vi "AUTOFOCUS_automatic_detection.vi"(0 "X array":dbl[](array[numeric]), 1 "QPD array":dbl[](array[numeric]), 2 "Stage type":string, 5 "QPD ref":T1, 7 "Slope":dbl, 9 "QPD":T1, 11 "error in":errorcluster, 12 "Search array":dbl[](array[numeric])) -> (3 "QPD array out":dbl[](array[numeric]), 4 "X array out":dbl[](array[numeric]), 6 "Cursor":cluster{"X":dbl, "Y":dbl}, 8 "Setpoint detected":bool, 10 "norm":dbl, 15 "error out":errorcluster)   [LabVIEW 2015]
uses:
  <vilib>/Analysis/_algsub.llb/Vector Norm Type.ctl
  <vilib>/Analysis/_algsub.llb/Real Vector Norm.vi
  <vilib>/Analysis/NI_AAL_SigProc.lvlib
  <vilib>/Analysis/NI_AALPro.lvlib
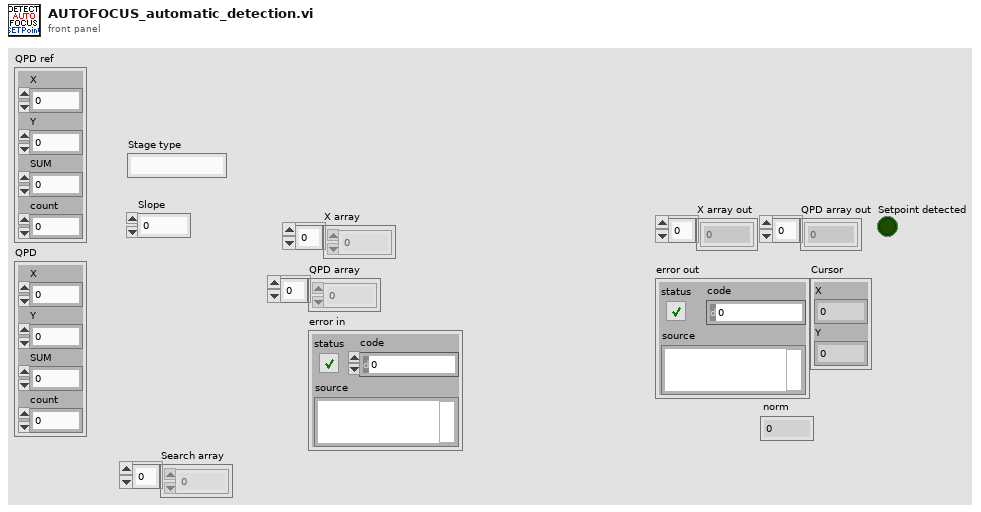
[diagram p1: front panel]
types:
  T1 = cluster{"X":sgl, "Y":sgl, "SUM":sgl, "count":u32}
  T2 = typedef "NI_AALPro.lvlib/Vector Norm Type.ctl" = u16
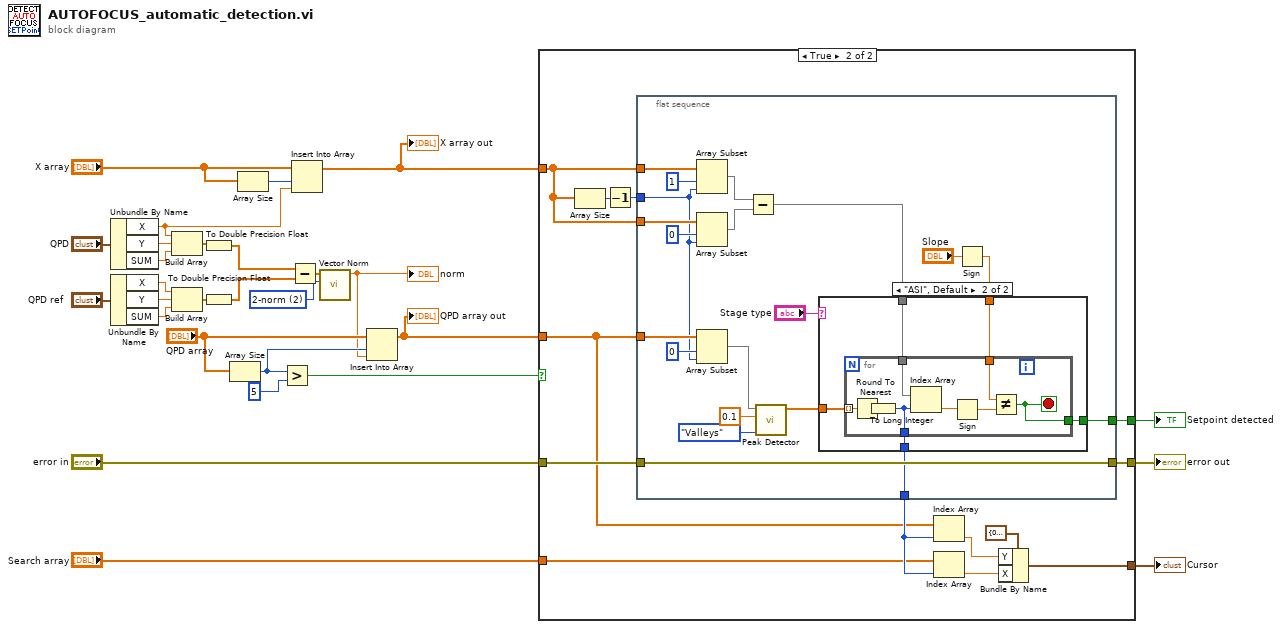
[diagram p0: block diagram]
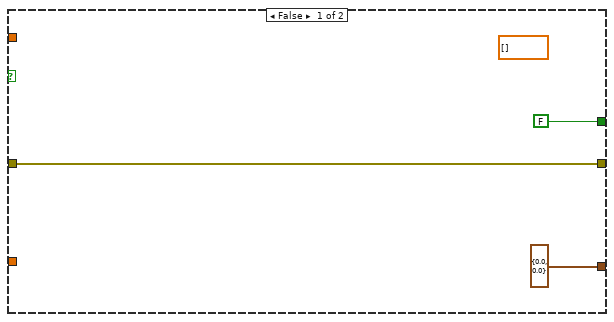
[diagram p2: hidden frame]
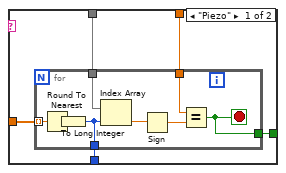
[diagram p3: hidden frame]
diagram:
  w18 = T2 2 items=["1-norm"=1, "2-norm"=2, "Inf-norm"=3, "-Inf-norm"=4, "User Defined"=5] ("norm type")
  n1 = Unbundle By Name("QPD") -> ("X"=w3:sgl, "Y"=w12:sgl, "SUM"=w11:sgl)
  n2 = Unbundle By Name("QPD ref") -> ("X"=w6:sgl, "Y"=w8:sgl, "SUM"=w9:sgl)
  n3 = Build Array(w3, w12, w11) -> (w10:sgl[])
  n4 = Build Array(w6, w8, w9) -> (w7:sgl[])
  n5 = To Double Precision Float(number=w10) -> (double precision float=w2:dbl[])
  n6 = To Double Precision Float(number=w7) -> (double precision float=w1:dbl[])
  n7 = Array Size(array="QPD array") -> (size(s)=w16:i32)
  n8 = Array Size(array="X array") -> (size(s)=w22:i32)
  n9 = Greater?(x=w16, y=5) -> (0:w27:bool)
  n10 = Subtract(x=w2, y=w1) -> (x-y=w19:dbl[])
  n11 = Insert Into Array(array="X array", index=w22, new element=w3) -> (w20:dbl[])
  "X array out" <- w20
  n12 = call-poly <vilib>:"Vector Norm.vi"("norm type"=w18, "Input Vector"=w19) -> ("norm"=w15:dbl)  [unwired: 8 in, 1 out]
  "norm" <- w15
  n13 = Insert Into Array(array="QPD array", index=w16, new element=w15) -> (w14:dbl[])
  "QPD array out" <- w14
  n14 = case shown="True" w27 {
    tunnel: "error in" -> [w31 w41]
    tunnel: [w31 w40] -> w24
    tunnel: "Search array" -> [_ w39]
    tunnel: [cluster{"X":dbl, "Y":dbl} {"X"=0.0, "Y"=0.0} ("Position") w35] -> w23
    tunnel: w20 -> [_ w34]
    tunnel: w14 -> [_ w33]
    tunnel: [FALSE w32] -> w13
    frame False {
      (unwired) dbl[] []
    }
    frame True {
      n15 = Array Size(array=w34) -> (size(s)=w42:i32)
      n16 = Decrement(x=w42) -> (x-1=w43:i32)
      n17 = flat-sequence {
        tunnel: [w48] -> w44
        tunnel: w33 -> [w54]
        tunnel: [w62] -> w40
        tunnel: w41 -> [w62]
        tunnel: w34 -> [w61]
        tunnel: w43 -> [w53]
        tunnel: w34 -> [w59]
        tunnel: [w46] -> w32
        frame #0 {
          n18 = Array Subset(array=w61, index=1, length=w53) -> (w57:dbl[])
          n19 = Array Subset(array=w59, index=0, length=w53) -> (w56:dbl[])
          n20 = Array Subset(array=w54, index=0, length=w53) -> (w47:dbl[])
          n21 = Subtract(x=w57, y=w56) -> (x-y=w51:dbl[])
          n22 = call <vilib>:"Peak Detector.vi"("peaks/valleys"=enum32{"Peaks", "Valleys"}."Valleys", "threshold"=0.1, "X"=w47) -> ("Locations"=w52:dbl[])  [unwired: 4 in, 4 out]
          n23 = Sign(1:"Slope") -> (0:w49:dbl)
          n24 = case shown="\"ASI\", Default" "Stage type" {
            tunnel: w52 -> [w69 w82]
            tunnel: w51 -> [w68 w81]
            tunnel: w49 -> [w67 w80]
            tunnel: [w66 w79] -> w48
            tunnel: [w65 w78] -> w46
            frame "Piezo" {
              n25 = for {
                tunnel: w69 -> [w77] mode=indexing
                tunnel: w68 -> [w75]
                tunnel: w67 -> [w72]
                tunnel: [w71] -> w66
                tunnel: [w70] -> w65
                stop <- w70 stop-if-true
                n26 = Round To Nearest(number=w77) -> (nearest integer value=w76:dbl)
                n27 = To Long Integer(number=w76) -> (32bit integer=w71:i32)
                n28 = Index Array(array=w75, index=w71) -> (element=w74:dbl)
                n29 = Sign(1:w74) -> (0:w73:dbl)
                n30 = Equal?(x=w72, y=w73) -> (x = y?=w70:bool)
              }
            }
            frame "ASI", Default {
              n31 = for {
                tunnel: w82 -> [w90] mode=indexing
                tunnel: w81 -> [w88]
                tunnel: w80 -> [w85]
                tunnel: [w84] -> w79
                tunnel: [w83] -> w78
                stop <- w83 stop-if-true
                n32 = Round To Nearest(number=w90) -> (nearest integer value=w89:dbl)
                n33 = To Long Integer(number=w89) -> (32bit integer=w84:i32)
                n34 = Index Array(array=w88, index=w84) -> (element=w87:dbl)
                n35 = Sign(1:w87) -> (0:w86:dbl)
                n36 = Not Equal?(x=w85, y=w86) -> (x != y?=w83:bool)
              }
            }
          }
        }
      }
      n37 = Index Array(array=w33, index=w44) -> (element=w37:dbl)
      n38 = Index Array(array=w39, index=w44) -> (element=w36:dbl)
      n39 = Bundle By Name(cluster=cluster{"X":dbl, "Y":dbl} {"X"=0.0, "Y"=0.0} ("Position"), "Y"=w37, "X"=w36) -> (w35:cluster{"X":dbl, "Y":dbl})
    }
  }
  "error out" <- w24
  "Cursor" <- w23
  "Setpoint detected" <- w13
